vi "Connection Put Signal.vi"(0 "Connection DVR in":refnum<data-value>, 5 "Data":refnum<data-value>, 7 "time":refnum<data-value>, 9 "Path in":string, 11 "error in (no error)":errorcluster) -> (4 "Connection DVR out":refnum<data-value>, 15 "error out":errorcluster)   [LabVIEW 2015, in "MDSplus.lvlib"]
uses:
  MDSplus.lvlib
  Classes/Data_Class/Data.lvclass
  Classes/Connection_Class/Connection.lvclass
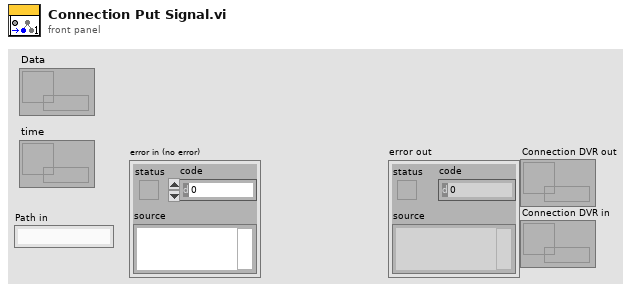
[diagram p1: front panel]
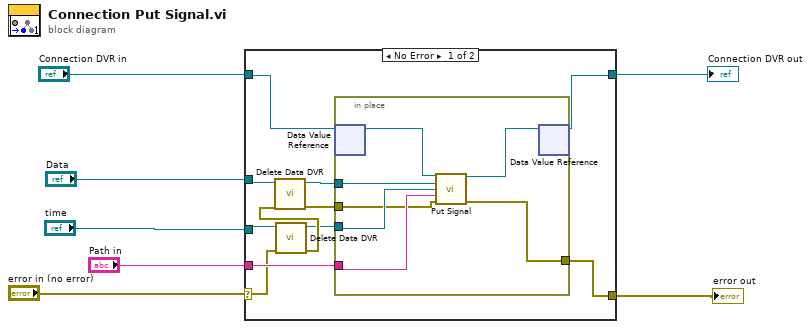
[diagram p0: block diagram]
diagram:
  n1 = case shown="No Error" "error in (no error)" {
    selector: "error in (no error)" -> [w14 w26]
    tunnel: "Connection DVR in" -> [w18 w27]
    tunnel: [w17 w27] -> w5
    tunnel: [w9 w26] -> w4
    tunnel: "Data" -> [w8 _]
    tunnel: "Path in" -> [w16 _]
    tunnel: "time" -> [w15 _]
    frame No Error {
      n2 = call "Delete Data DVR.vi"("error in (no error)"=w14, "Data DVR in"=w15) -> ("error out"=w13:errorcluster, "Data out"=w10:refnum<class "Data.lvclass">)  [unwired: 8 in]
      n3 = call "Delete Data DVR.vi"("error in (no error)"=w13, "Data DVR in"=w8) -> ("error out"=w12:errorcluster, "Data out"=w11:refnum<class "Data.lvclass">)  [unwired: 8 in]
      n4 = in-place {
        in-place-border: w16 -> [w23]
        in-place-border: w12 -> [w22]
        in-place-border: w11 -> [w24]
        in-place-border: w10 -> [w25]
        in-place-border: [w21] -> w9
        n5 = in-place-dvr #1(w18) -> (w20:refnum<class "Connection.lvclass">)  [unwired: 1 out]
        n6 = call "Put Signal.vi"("Connection in"=w20, "Data"=w24, "Time"=w25, "Path in"=w23, "error in (no error)"=w22) -> ("Connection out"=w19:refnum<class "Connection.lvclass">, "error out"=w21:errorcluster)  [unwired: 9 in]
        n7 = in-place-dvr #1(w19) -> (w17:refnum<data-value>)  [unwired: 1 out]
      }
    }
    frame Error {
    }
  }
  "error out" <- w4
  "Connection DVR out" <- w5
